vi "Instance FG.vi"(8 "error in (no error)":errorcluster, 11 "App in":refnum<class "App.lvclass">) -> (0 "error out":errorcluster, 3 "App out":refnum<class "App.lvclass">)   [LabVIEW 2020, in "PicoG-App.lvlib" / "App.lvclass"]
uses:
  App.lvclass
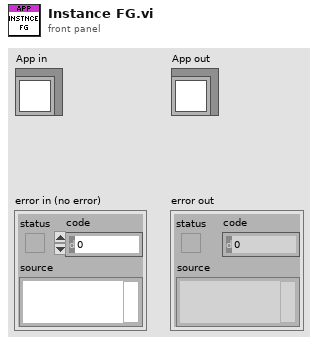
[diagram p1: front panel]
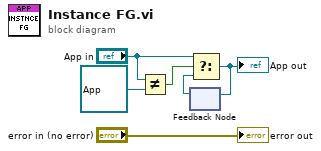
[diagram p0: block diagram]
diagram:
  n1 = Not Equal?(x="App in", y=refnum<class "App.lvclass"> refnum ("App in")) -> (x != y?=w1:bool)
  n2 = feedback #1() -> (w4:refnum<class "App.lvclass">)  [unwired: 1 in]
  n3 = Select(t="App in", s=w1, f=w4) -> (s? t:f=w5:refnum<class "App.lvclass">)
  "App out" <- w5
  n4 = feedback-in #1(w5) -> ()
  "error out" <- "error in (no error)"
